vi "SVT Gain (Frequency) (1 Ch).vi"(0 "complex spectrum":T9={"complex spectrum response"={"f0"=0.0, "df"=1.0, "complex spectrum"=[]}, "spectrum info"={"channel name"="", "description"="", "x-axis units"=0, "spectral info"={"spectrum type"=enum."Power [Magnitude^2]", "linear/dB"=enum."linear", "window"=0, "window size"=0, "FFT size"=0}, "engineering units"=0, "custom label"="", "dB reference [EU]"=0.0, "peak units"=enum."rms", "weighting filter"=0, "spectral density?"=FALSE, "unit label"="", "spectrum skewed?"=FALSE, "complimentary spectrum units"=enum."none"}} {"spectrum info"."x-axis units" items=["Time (s)"=0, "Frequency-CB (Hz)"=1, "Frequency-CPB (Hz)"=1248, "Frequency-Arbitrary (Hz)"=2357, "Quefrency (s)"=2, "Revolutions (rev)"=3, "Order"=4, "Speed (RPM)"=11, "Speed (rad/s)"=21, "Index"=65535]; "spectrum info"."weighting filter" items=["Linear", "A-weighting", "B-weighting", "C-weighting", "ITU-R 468-4", "Dolby", "CCITT", "C-message", "Wb", "Wc", "Wd", "We", "Wf", "Wh", "Wj", "Wk", "Wm", "AES17 20 kHz lowpass", "AES17 40 kHz lowpass", "AES17 20 kHz highpass", "AES17 40 kHz highpass"]; "spectrum info"."dB reference [EU]" format="%.2f"; "spectrum info"."engineering units" items=["custom..."=0, "V"=1, "A"=21, "C"=30, "pC"=31, "s"=32, "-"=29, "Pa"=2, "N"=20, "g"=3, "m/s^2"=4, "m/s"=5, "m"=6, "mm/s"=12, "mm"=13, "micron/s"=14, "micron"=15, "in/s^2"=7, "in/s"=8, "in"=9, "mil/s"=10, "mil"=11, "rad/s^2"=16, "rad/s"=17, "rad"=18, "deg/s^2"=26, "deg/s"=27, "deg"=28, "RPM"=22, "cycle/s^2"=23, "Hz"=24, "cycle"=25, "strain"=19]; "spectrum info"."spectral info"."window" items=["None "=0, "Hanning"=1, "Hamming"=2, "Blackman-Harris"=3, "Exact Blackman"=4, "Blackman"=5, "Flat Top"=6, "4 Term B-Harris "=7, "7 Term B-Harris"=8, "Low Sidelobe"=9, "Force - Exponential"=10, "Gaussian"=62]; "complex spectrum response"."complex spectrum" format="%.2f"; "complex spectrum response"."df" format="%.2f"; "complex spectrum response"."f0" format="%.2f"}, 3 "advanced span [Hz]":dbl=-1.0 format="%.2f", 5 "error in (no error)":errorcluster, 6 "desired units":T2, 7 "amplitude [EU peak]":dbl=1.0 format="%.2f", 9 "expected fundamental \nfrequency [Hz]":dbl=-1.0 format="%.2f") -> (11 "detected fundamental\nfrequency [Hz]":dbl=nan format="%.2f", 12 "unit labels":T1, 13 "detected fundamental\namplitude":dbl=nan format="%.2f", 14 "dup complex spectrum":T9={"complex spectrum response"={"f0"=0.0, "df"=1.0, "complex spectrum"=[]}, "spectrum info"={"channel name"="", "description"="", "x-axis units"=0, "spectral info"={"spectrum type"=enum."Power [Magnitude^2]", "linear/dB"=enum."linear", "window"=0, "window size"=0, "FFT size"=0}, "engineering units"=0, "custom label"="", "dB reference [EU]"=0.0, "peak units"=enum."rms", "weighting filter"=0, "spectral density?"=FALSE, "unit label"="", "spectrum skewed?"=FALSE, "complimentary spectrum units"=enum."none"}} {"spectrum info"."x-axis units" items=["Time (s)"=0, "Frequency-CB (Hz)"=1, "Frequency-CPB (Hz)"=1248, "Frequency-Arbitrary (Hz)"=2357, "Quefrency (s)"=2, "Revolutions (rev)"=3, "Order"=4, "Speed (RPM)"=11, "Speed (rad/s)"=21, "Index"=65535]; "spectrum info"."weighting filter" items=["Linear", "A-weighting", "B-weighting", "C-weighting", "ITU-R 468-4", "Dolby", "CCITT", "C-message", "Wb", "Wc", "Wd", "We", "Wf", "Wh", "Wj", "Wk", "Wm", "AES17 20 kHz lowpass", "AES17 40 kHz lowpass", "AES17 20 kHz highpass", "AES17 40 kHz highpass"]; "spectrum info"."dB reference [EU]" format="%.2f"; "spectrum info"."engineering units" items=["custom..."=0, "V"=1, "A"=21, "C"=30, "pC"=31, "s"=32, "-"=29, "Pa"=2, "N"=20, "g"=3, "m/s^2"=4, "m/s"=5, "m"=6, "mm/s"=12, "mm"=13, "micron/s"=14, "micron"=15, "in/s^2"=7, "in/s"=8, "in"=9, "mil/s"=10, "mil"=11, "rad/s^2"=16, "rad/s"=17, "rad"=18, "deg/s^2"=26, "deg/s"=27, "deg"=28, "RPM"=22, "cycle/s^2"=23, "Hz"=24, "cycle"=25, "strain"=19]; "spectrum info"."spectral info"."window" items=["None "=0, "Hanning"=1, "Hamming"=2, "Blackman-Harris"=3, "Exact Blackman"=4, "Blackman"=5, "Flat Top"=6, "4 Term B-Harris "=7, "7 Term B-Harris"=8, "Low Sidelobe"=9, "Force - Exponential"=10, "Gaussian"=62]; "complex spectrum response"."complex spectrum" format="%.2f"; "complex spectrum response"."df" format="%.2f"; "complex spectrum response"."f0" format="%.2f"}, 16 "gain":dbl=nan format="%.2f", 19 "error out":errorcluster)   [LabVIEW 2017, in "SoundVib_SingleTone.lvlib"]
doc: "Computes the gain of a channel based on <B>scaled signal</B> and <B>amplitude</B> at the fundamental frequency. This VI returns the detected fundamental frequency, detected fundamental amplitude, and gain. This VI does not maintain state internally; you can use this VI in a loop to process multiple blocks. Wire data to the <B>scaled signal [EU]</B> input to determine the polymorphic instance to use or manually select the instance."
uses:
  <vilib>/addons/Sound and Vibration/svt_Single Tone Measurements/SoundVib_SingleTone.lvlib
  <vilib>/addons/_NISVFA/_Shared subVIs/Controls/svc_Spectrum Info.ctl
  <vilib>/addons/_NISVFA/_Shared subVIs/Controls/svc_X-Axis Units.ctl
  <vilib>/addons/_NISVFA/_Shared subVIs/Controls/svc_Spectrum Type.ctl
  <vilib>/addons/_NISVFA/_Shared subVIs/Controls/svc_Engineering Units Text Ring.ctl
  <vilib>/addons/_NISVFA/_Shared subVIs/Controls/svc_Weighting Filter Text Ring.ctl
  <vilib>/addons/_NISVFA/_Shared subVIs/Controls/svc_Complimentary Spectrum Units.ctl
  <vilib>/addons/Sound and Vibration/svt_Distortion/SoundVib_Distortion.lvlib
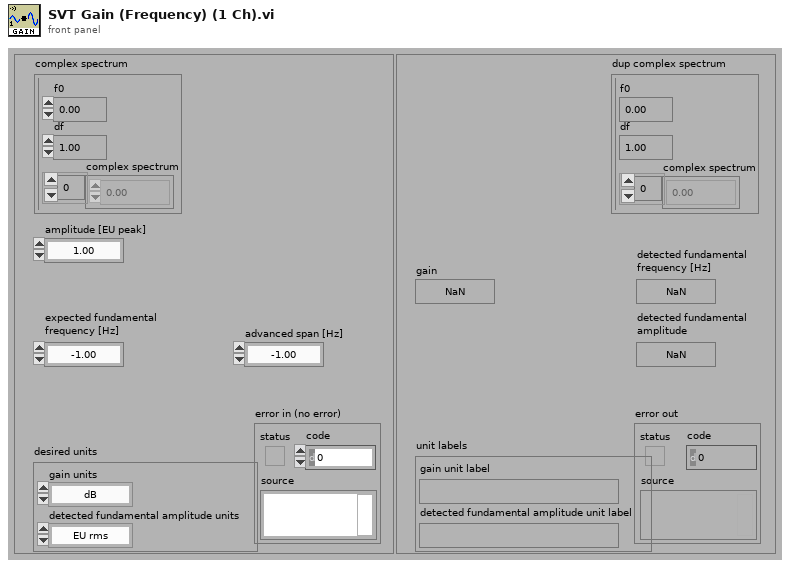
[diagram p1: front panel]
types:
  T1 = cluster{"gain unit label":string, "detected fundamental amplitude unit label":string}
  T2 = cluster{"gain units":enum16{"dB", "linear ratio"}, "detected fundamental amplitude units":enum16{"EU rms", "EU peak", "EU peak-peak"}}
  T3 = typedef "svc_Spectrum Info.ctl" = cluster{"channel name":string, "description":string, "x-axis units":T4, "spectral info":cluster{"spectrum type":T5, "linear/dB":enum16{"linear", "dB"}, "window":u16, "window size":i32, "FFT size":i32}, "engineering units":T6, "custom label":string, "dB reference [EU]":dbl, "peak units":enum16{"rms", "peak", "peak-peak"}, "weighting filter":T7, "spectral density?":bool, "unit label":string, "spectrum skewed?":bool, "complimentary spectrum units":T8}
  T4 = typedef "svc_X-Axis Units.ctl" = u16
  T5 = typedef "svc_Spectrum Type.ctl" = enum16{"FFT Spectrum [complex]", "Amplitude [Magnitude]", "Power [Magnitude^2]", "Cross Spectrum [complex]", "Frequency Response [Complex]"}
  T6 = typedef "svc_Engineering Units Text Ring.ctl" = u16
  T7 = typedef "svc_Weighting Filter Text Ring.ctl" = u16
  T8 = typedef "svc_Complimentary Spectrum Units.ctl" = enum16{"none", "radians", "degrees", "cycles", "imaginary"}
  T9 = cluster{"complex spectrum response":cluster{"f0":dbl, "df":dbl, "complex spectrum":cdb[]}, "spectrum info":T3}
  T10 = enum32{"none", "input signal", "detected signal", "residual signal"}
  T11 = cluster{"unit label":string, "unit label":string}
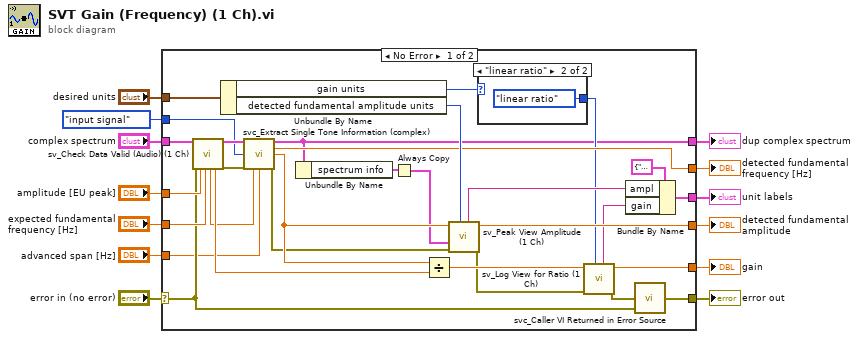
[diagram p0: block diagram]
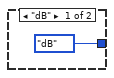
[diagram p2: hidden frame]
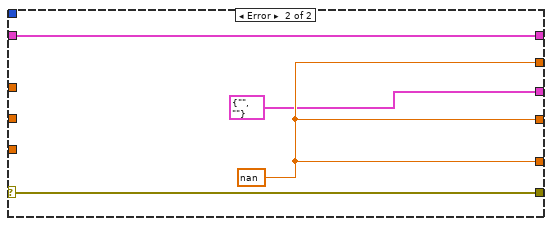
[diagram p3: hidden frame]
diagram:
  n1 = case shown="No Error" "error in (no error)" {
    selector: "error in (no error)" -> [w23 w49]
    tunnel: "complex spectrum" -> [w32 w46]
    tunnel: "expected fundamental \nfrequency [Hz]" -> [w33 _]
    tunnel: "amplitude [EU peak]" -> [w35 _]
    tunnel: [w40 w48] -> w11
    tunnel: [w27 w48] -> w9
    tunnel: [w39 w48] -> w8
    tunnel: "desired units" -> [w43 _]
    tunnel: [w37 T11 {"unit label"="", "unit label"=""}] -> w6
    tunnel: [w36 w49] -> w10
    tunnel: [w17 w46] -> w3
    tunnel: T10."input signal" ("export signals") -> [w15 _]
    tunnel: "advanced span [Hz]" -> [w14 _]
    frame No Error {
      n2 = call <vilib>:"sv_Check Data Valid (Audio) (1 Ch).vi"("complex spectrum"=w32, "error in (no error)"=w23, "amplitude"=w35, "expected fundamental frequency [Hz]"=w33) -> ("dup expected fundamental frequency [Hz]"=w24:dbl, "dup amplitude"=w34:dbl, "complex spectrum"=w26:T9, "error out"=w25:errorcluster)  [unwired: 8 in, 4 out]
      n3 = Unbundle By Name(w43) -> ("gain units"=w22:enum16{"dB", "linear ratio"}, "detected fundamental amplitude units"=w42:enum16{"EU rms", "EU peak", "EU peak-peak"})
      n4 = call <vilib>:"svc_Extract Single Tone Information (complex).vi"("complex spectrum"=w26, "export signals"=w15, "error in"=w25, "approximate frequency [Hz]"=w24, "advanced span [Hz]"=w14) -> ("complex spectrum"=w17:T9, "frequency [Hz]"=w27:dbl, "amplitude [EU pk]"=w28:dbl, "error out"=w16:errorcluster)  [unwired: 5 in, 2 out]
      n5 = Unbundle By Name(w17) -> ("spectrum info"=w31:T3)
      n6 = Always Copy(1:w31) -> (0:w20:T3)
      n7 = Divide(x=w28, y=w34) -> (x/y=w41:dbl)
      n8 = call <vilib>:"sv_Peak View Amplitude (1 Ch).vi"("peak units"=w42, "error in (no error)"=w16, "spectrum info"=w20, "peak amplitude [EU pk]"=w28) -> ("error out"=w30:errorcluster, "converted peak amplitude"=w39:dbl, "unit label"=w38:string)  [unwired: 5 in]
      n9 = case shown="\"linear ratio\"" w22 {
        tunnel: [enum16{"dB", "linear ratio", "%"}."dB" ("ratio units") enum16{"dB", "linear ratio", "%"}."linear ratio" ("ratio units")] -> w21
        frame "dB" {
        }
        frame "linear ratio" {
        }
      }
      n10 = call <vilib>:"sv_Log View for Ratio (1 Ch).vi"("ratio units"=w21, "error in (no error)"=w30, "linear ratio"=w41) -> ("error out"=w29:errorcluster, "converted ratio"=w40:dbl, "unit label"=w18:string)  [unwired: 6 in]
      n11 = Bundle By Name(cluster=cluster{"gain":string, "ampl":string} {"gain"="", "ampl"=""} ("unit labels"), "ampl"=w38, "gain"=w18) -> (w37:cluster{"gain":string, "ampl":string})
      n12 = call <vilib>:"svc_Caller VI Returned in Error Source.vi"("warning input to caller"=w23, "error in (no error)"=w29) -> ("error out"=w36:errorcluster)  [unwired: 3 in]
    }
    frame Error {
      w48 = nan
    }
  }
  "gain" <- w11
  "error out" <- w10
  "dup complex spectrum" <- w3
  "detected fundamental\nfrequency [Hz]" <- w9
  "detected fundamental\namplitude" <- w8
  "unit labels" <- w6
